vi "Send Message.vi"(8 "error in (no error)":errorcluster, 10 "Message":refnum<class "tBSONDocument.lvclass">, 11 "tWorkerTCPConnection in":refnum<class "tWorkerTCPConnection.lvclass">) -> (0 "error out":errorcluster, 3 "tWorkerTCPConnection out":refnum<class "tWorkerTCPConnection.lvclass">)   [LabVIEW 2014, in "tWorkerTCPConnection.lvlib" / "tWorkerTCPConnection.lvclass"]
uses:
  tWorkerTCPConnection.lvclass
  BSON/tBSONDocument/tBSONDocument.lvclass
  <vilib>/ActorFramework/Actor/Actor.lvclass/Actor.ctl
  tWorkerTCPConnection.lvclass/tWorkerTCPConnection.ctl
  tWorkerController/msgs/TCP Command Sent Msg/TCP Command Sent Msg.lvclass/TCP Command Sent Msg.ctl
  <vilib>/ActorFramework/Message Enqueuer/Message Enqueuer.lvclass/Message Enqueuer.ctl
  <vilib>/ActorFramework/Message Enqueuer/Enqueue.vi
  <vilib>/ActorFramework/Message Priority Queue/Priority Enqueue.vi
  tWorkerController/msgs/TCP Command Sent Msg/TCP Command Sent Msg.lvclass
  <vilib>/ActorFramework/Actor/Actor.lvclass
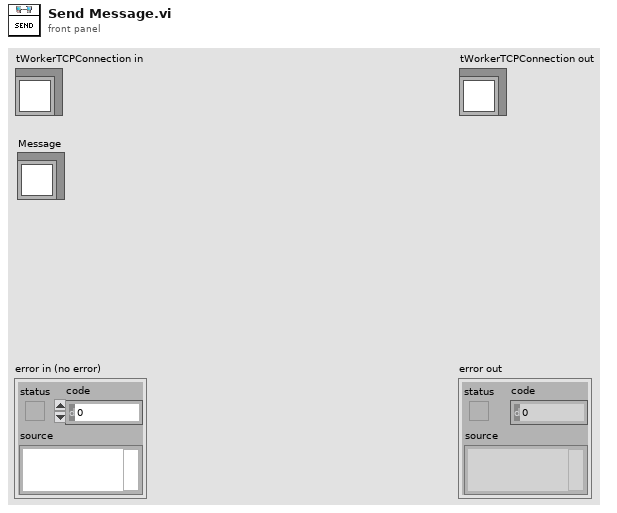
[diagram p1: front panel]
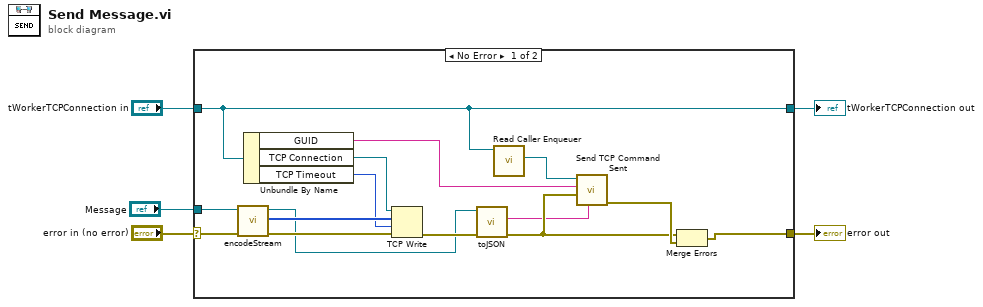
[diagram p0: block diagram]
diagram:
  n1 = case shown="No Error" "error in (no error)" {
    selector: "error in (no error)" -> [w20 w22]
    tunnel: [w10 w22] -> w4
    tunnel: [w14 w21] -> w2
    tunnel: "tWorkerTCPConnection in" -> [w14 w21]
    tunnel: "Message" -> [w19 _]
    frame No Error {
      n2 = call "encodeStream.vi"("error in (no error)"=w20, "tBSONDocument in"=w19) -> ("error out"=w18:errorcluster, "Byte Data"=w17:u8[], "tBSONDocument out"=w7:refnum<class "tBSONDocument.lvclass">)  [unwired: 7 in]
      n3 = Unbundle By Name(w14) -> ("GUID"=w12:string, "TCP Connection"=w16:refnum<k5>, "TCP Timeout"=w15:i32)
      n4 = TCP Write(connection ID=w16, data in=w17, error in (no error)=w18, 9:w15) -> (error out=w9:errorcluster)  [unwired: 2 out]
      n5 = call-dynamic "toJSON.vi"("error in (no error)"=w9, "tBSONDocument in"=w7) -> ("error out"=w8:errorcluster, "JSON"=w6:string)  [unwired: 7 in, 1 out]
      n6 = call <vilib>:"Read Caller Enqueuer.vi"("Actor"=w14) -> ("Caller Enqueuer"=w13:refnum<class "Message Enqueuer.lvclass">)  [unwired: 10 in]
      n7 = call "Send TCP Command Sent.vi"("Message"=w6, "Sending Error"=w8, "GUID"=w12, "Message Enqueuer"=w13) -> ("error out"=w11:errorcluster)  [unwired: 6 in, 1 out]
      n8 = Merge Errors(w8, w11) -> (w10:errorcluster)
    }
    frame Error {
    }
  }
  "error out" <- w4
  "tWorkerTCPConnection out" <- w2
